vi "P9P14_Temp_open_queue.vi"(8 "error in (no error)":errorcluster) -> (0 "error out":errorcluster, 2 "queue out":refnum<queue>)   [LabVIEW 2019]
uses:
  PPMS/P9P14-TCluster-Control.ctl
  Global/Global Variables/Queues_global.vi
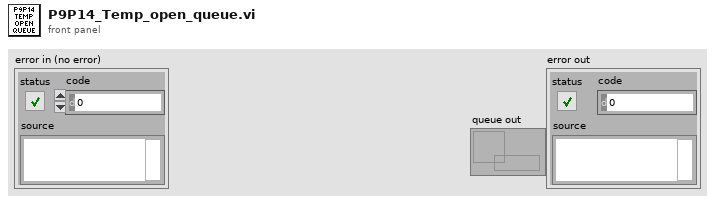
[diagram p1: front panel]
types:
  T1 = typedef "P9P14-TCluster-Control.ctl" = cluster{"Setpoint":dbl, "Rate":dbl, "Approach":u16, "Set":bool, "Autoshutdown":bool}
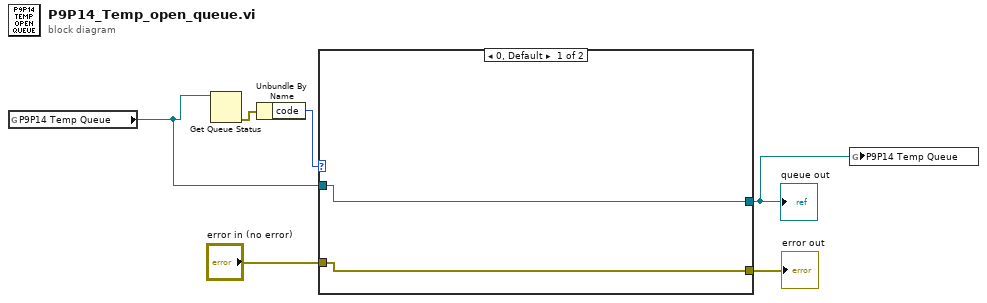
[diagram p0: block diagram]
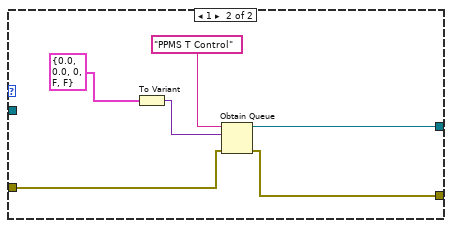
[diagram p2: hidden frame]
diagram:
  n1 = global read "Queues_global.vi" "P9P14 Temp Queue"() -> (w4:refnum<queue>)
  n2 = Get Queue Status(queue=w4) -> (error out=w6:errorcluster)  [unwired: 2 in, 7 out]
  n3 = Unbundle By Name(w6) -> ("code"=w5:i32)
  n4 = case shown="0, Default" w5 {
    tunnel: w4 -> [w8 _]
    tunnel: [w7 w14] -> w3
    tunnel: "error in (no error)" -> [w7 w13]
    tunnel: [w8 w9] -> w1
    frame 0, Default {
    }
    frame 1 {
      n5 = To Variant(anything=T1 {"Setpoint"=0.0, "Rate"=0.0, "Approach"=0, "Set"=FALSE, "Autoshutdown"=FALSE} ("P9-P14 T-Cluster -Control")) -> (Variant=w11:variant)
      n6 = Obtain Queue(name (unnamed)="PPMS T Control", element data type=w11, error in (no error)=w13) -> (queue out=w9:refnum<queue>, error out=w14:errorcluster)  [unwired: 2 in, 1 out]
    }
  }
  "error out" <- w3
  "queue out" <- w1
  n7 = global write "Queues_global.vi" "P9P14 Temp Queue"(w1) -> ()
